vi "SimpleEndpointController.vi"(0 "error in":errorcluster, 2 "Side":T1=enum."right", 3 "Controls":T2={"Rotation"=-42.91139240506329, "Distance"=17.78481012658228, "Wrist"=-20.886075949367083, "Height"=0.25316455696202533, "Hand Orientation"=enum."Down"} {"Height" scale=-10.0..10.0; "Wrist" scale=-90.0..90.0; "Distance" scale=10.0..25.0; "Rotation" scale=-60.0..60.0}, 4 "node":string) -> (1 "error out":errorcluster)   [LabVIEW 2015]
uses:
  ROS/Code/SubVIs/BaxterArmsSmall.ctl
  ROS/Code/SubVIs/BaxterSide.ctl
  ROS/Code/SubVIs/JointMode.ctl
panel:
  in  "Start":T3={"Elbow 0"=0.0, "Elbow 1"=55.8123726628928, "Shoulder 0"=0.0, "Shoulder 1"=-28.952431226064945, "Wrist 0"=0.0, "Wrist 1"=63.14005856317215, "Wrist 2"=0.0}
  out "Arm Angles (degrees)":T3={"Elbow 0"=0.0, "Elbow 1"=104.42629473516128, "Shoulder 0"=-42.91139240506329, "Shoulder 1"=-55.575297908284846, "Wrist 0"=0.0, "Wrist 1"=41.14900317312356, "Wrist 2"=-20.886075949367083}
  in  "d 4":dbl=10.0
  in  "d 3":dbl=15.0
  in  "d 2":dbl=14.0
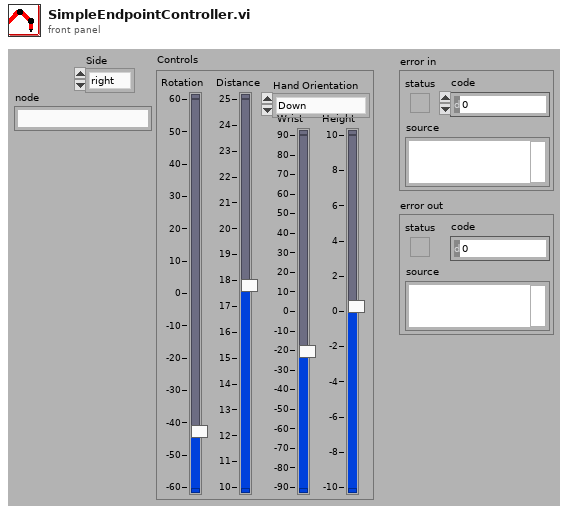
[diagram p1: front panel]
types:
  T1 = typedef "BaxterSide.ctl" = enum16{"left", "right"}
  T2 = cluster{"Rotation":dbl, "Distance":dbl, "Wrist":dbl, "Height":dbl, "Hand Orientation":enum16{"Down", "Flat"}}
  T3 = typedef "BaxterArmsSmall.ctl" = cluster{"Elbow 0":dbl, "Elbow 1":dbl, "Shoulder 0":dbl, "Shoulder 1":dbl, "Wrist 0":dbl, "Wrist 1":dbl, "Wrist 2":dbl}
  T4 = typedef "JointMode.ctl" = u8
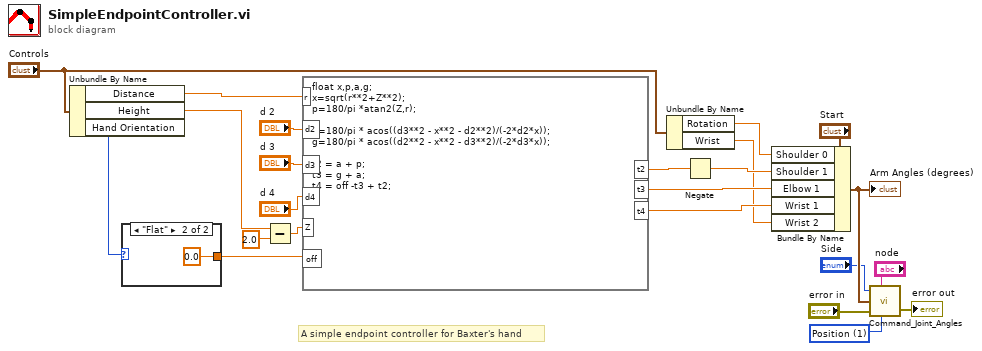
[diagram p0: block diagram]
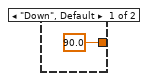
[diagram p2: hidden frame]
diagram:
  w6 = T4 1 items=["Position"=1, "Velocity"=2, "Effort"=3] ("Mode")
  # "A simple endpoint controller for Baxter's hand"
  n1 = Unbundle By Name("Controls") -> ("Distance"=w12:dbl, "Height"=w11:dbl, "Hand Orientation"=w10:enum16{"Down", "Flat"})
  n2 = case shown="\"Flat\"" w10 {
    tunnel: [90.0 ("y") 0.0 ("y")] -> w2
    frame "Down", Default {
    }
    frame "Flat" {
    }
  }
  n3 = Subtract(x=w11, y=2.0) -> (x-y=w13:dbl)
  n4 = formula code="float x,p,a,g;\nx=sqrt(r**2+Z**2);\np=180/pi *atan2(Z,r);\n\na=180/pi * acos((d3**2 - x**2 - d2**2)/(-2*d2*x));\ng=180/pi * acos((d2**2 - x**2 - d3**2)/(-2*d3*x));\n\nt2 = a + p;\nt3 = g + a;\nt4 = off -t3 + t2;"("r"=w12, "d2"="d 2", "d3"="d 3", "d4"="d 4", "Z"=w13, "off"=w2) -> ("t2"=w18:dbl, "t3"=w17:dbl, "t4"=w16:dbl)
  n5 = Unbundle By Name("Controls") -> ("Rotation"=w8:dbl, "Wrist"=w7:dbl)
  n6 = Negate(x=w18) -> (-x=w15:dbl)
  n7 = Bundle By Name(cluster="Start", "Shoulder 0"=w8, "Shoulder 1"=w15, "Elbow 1"=w17, "Wrist 1"=w16, "Wrist 2"=w7) -> (w22:T3)
  "Arm Angles (degrees)" <- w22
  n8 = call "Command_Joint_Angles.vi"("Side"="Side", "node"="node", "Arm Angles (degrees)"=w22, "error in"="error in", "Mode"=w6) -> ("error out"=→"error out":errorcluster)  [unwired: 1 in]
